vi "CreateCodeCoverage.vi"(5 "CodeCoverage in":refnum<class "CodeCoverage.lvclass">, 8 "error in (no error)":errorcluster) -> (0 "error out":errorcluster, 3 "CodeCoverage out":refnum<class "CodeCoverage.lvclass">)   [LabVIEW 2019, in "CodeCoverage.lvclass"]
uses:
  CodeCoverage.lvclass
  CodeCoverage.lvclass/CodeCoverage.ctl
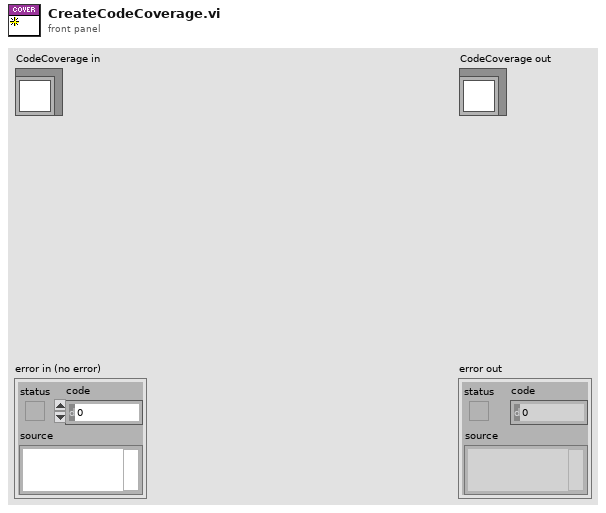
[diagram p1: front panel]
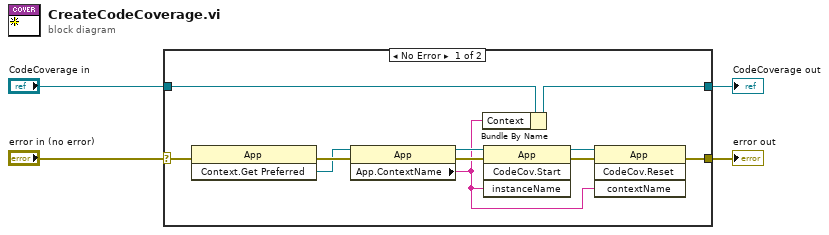
[diagram p0: block diagram]
diagram:
  n1 = case shown="No Error" "error in (no error)" {
    selector: "error in (no error)" -> [w9 w17]
    tunnel: [w7 w17] -> w3
    tunnel: [w10 w16] -> w1
    tunnel: "CodeCoverage in" -> [w15 w16]
    frame No Error {
      n2 = invoke class="App" method="Context.Get Preferred"(error in=w9) -> (error out=w14:errorcluster, "Get Preferred Context"=w11:refnum<vi>)  [unwired: 2 in, 1 out]
      n3 = property class="App"(reference=w11, error in=w14) -> (reference out=w12:refnum<vi>, error out=w13:errorcluster, "App.ContextName"=w5:string)
      n4 = Bundle By Name(cluster=w15, "Context"=w5) -> (w10:refnum<class "CodeCoverage.lvclass">)
      n5 = invoke class="App" method="CodeCov.Start"(reference=w12, error in=w13, "instanceName"=w5) -> (reference out=w6:refnum<vi>, error out=w8:errorcluster)  [unwired: 1 in, 2 out]
      n6 = invoke class="App" method="CodeCov.Reset"(reference=w6, error in=w8, "contextName"=w5) -> (error out=w7:errorcluster)  [unwired: 1 in, 3 out]
    }
    frame Error {
    }
  }
  "error out" <- w3
  "CodeCoverage out" <- w1
